vi "Error Log Example.vi"(3 "Send Error":bool, 4 "Erase":bool, 5 "Error Message":string="Error log message.", 6 "Show Console":bool, 7 "Error Level":T2(ring), 9 "Name":string(combo), 10 "Logger Display Format":T1=enum."PlainText.INI", 11 "Logger Name":string="Logger Example") -> ()   [LabVIEW 2018]
uses:
  <vilib>/BenjaminR/Error Log/Serializer/Type Defs/Display Format.ctl
  <vilib>/BenjaminR/Error Log/Handler.File.Text/Handler.File.Text.lvclass
  D:/Program Files (x86)/National Instruments/LabVIEW 2018/vi.lib/BenjaminR/Error Log/Handler/Handler.lvclass
  <vilib>/BenjaminR/Error Log/Handler.UserEvent.Console/Handler.UserEvent.Console.lvclass
  <userlib>/_OpenG.lib/file/file.llb/File Exists - Scalar__ogtk.vi
  <vilib>/BenjaminR/Error Log/Logger/Logger.lvclass
  <vilib>/BenjaminR/Error Log/Serializer/Serializer.lvlib
panel:
  in  "error in (no error)":errorcluster caption="错误输入（无错误）"
  in  "Error":errorcluster={"status"=TRUE, "code"=5000, "source"="My Error Code"}
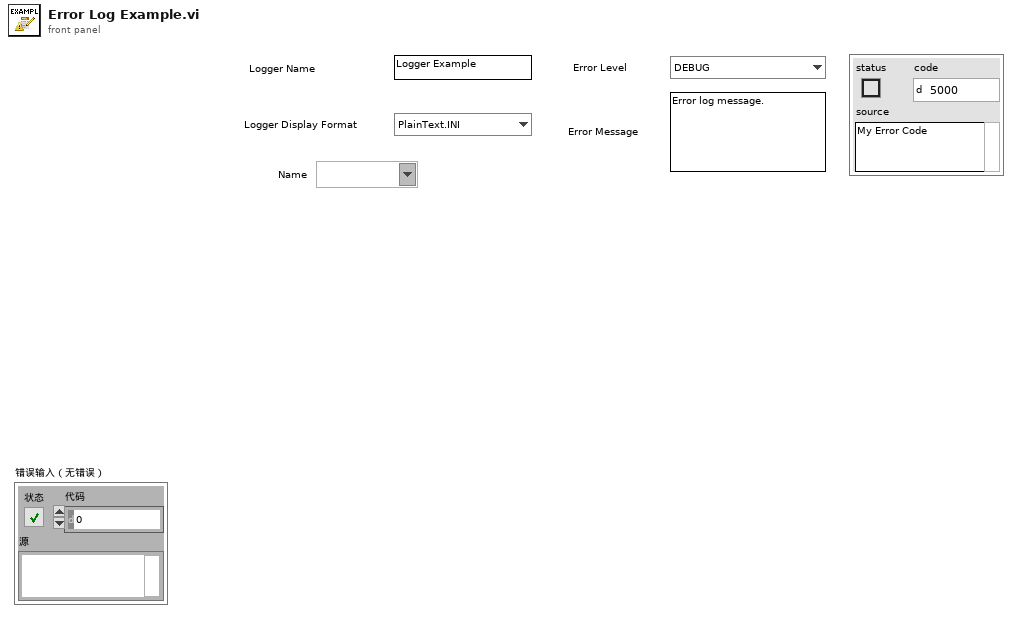
[diagram p1: front panel]
types:
  T1 = typedef "Serializer.lvlib/Display Format.ctl" = enum16{"PlainText", "PlainText.INI", "XML", "JSON"}
  T2 = enum16{"DEBUG", "INFO", "WARNING", "ERROR", "CRITICAL"}
  T3 = enum16{"open", "replace", "create", "open or create", "replace or create", "replace or create with confirmation"}
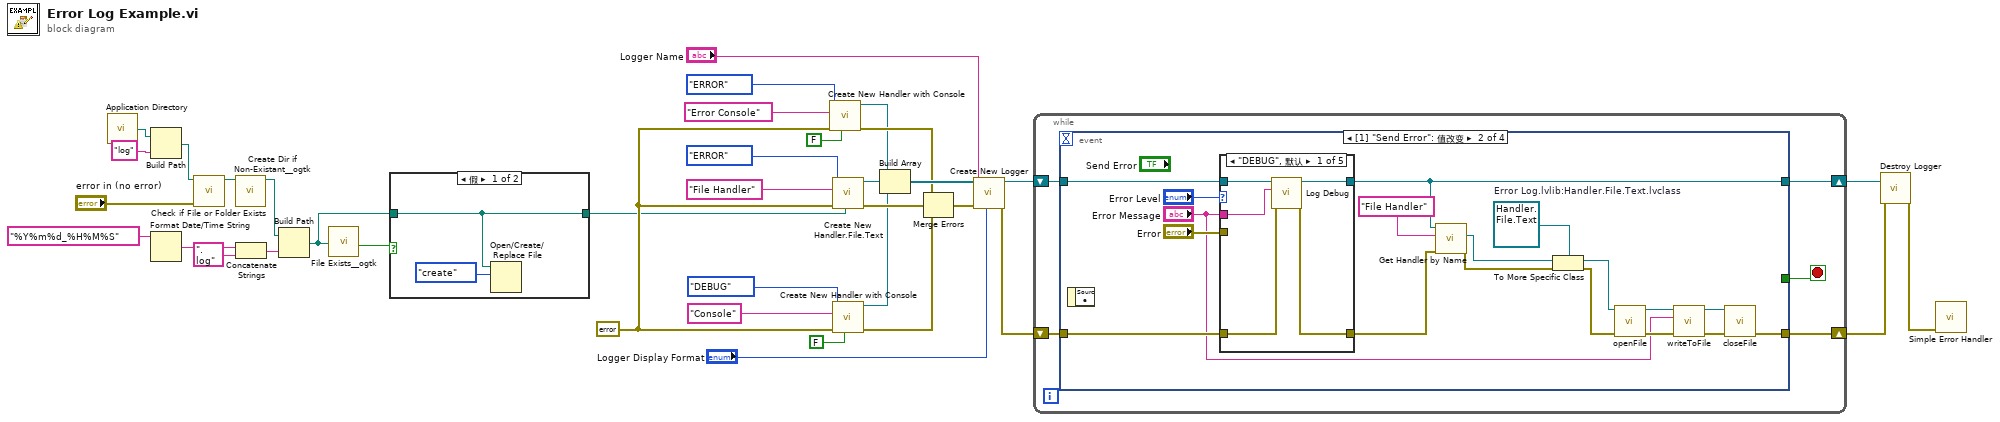
[diagram p0: block diagram]
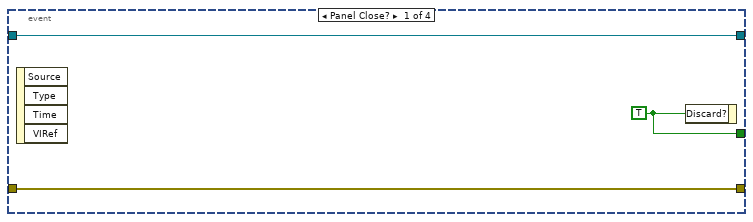
[diagram p3: hidden frame]
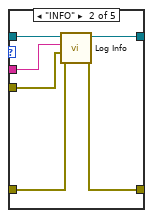
[diagram p4: hidden frame]
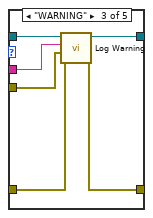
[diagram p5: hidden frame]
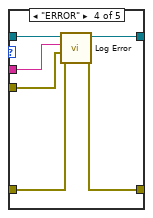
[diagram p6: hidden frame]
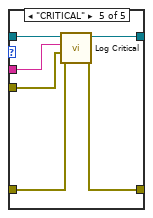
[diagram p7: hidden frame]
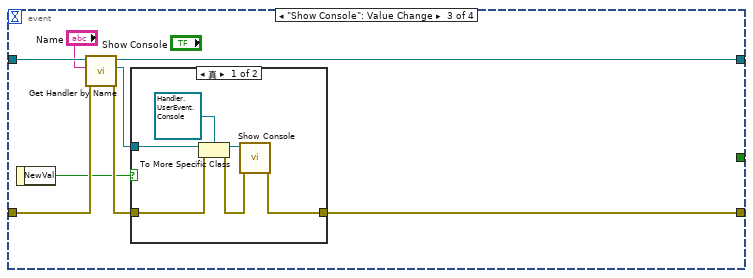
[diagram p8: hidden frame]
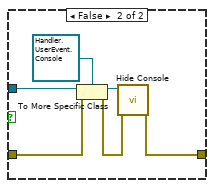
[diagram p9: hidden frame]
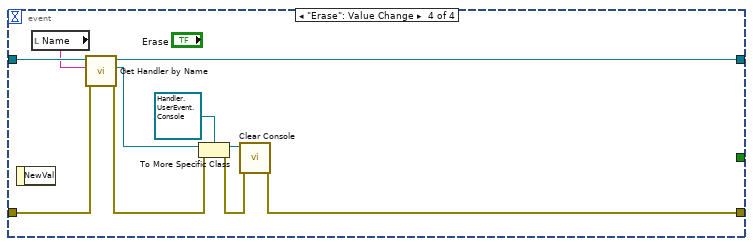
[diagram p10: hidden frame]
diagram:
  w16 = errorcluster {"status"=FALSE, "code"=0, "source"=""} ("error in (no error)")
  n1 = call <vilib>:"Application Directory.vi"() -> ("Application Directory"=w15:path)
  n2 = Build Path(base path=w15, name or relative path="log") -> (appended path=w13:path)
  n3 = Format Date/Time String(time format string (%c)="%Y%m%d_%H%M%S" ("时间格式字符串(%c)")) -> (date/time string=w8:string)  [unwired: 2 in]
  n4 = call <vilib>:"Check if File or Folder Exists.vi"("error in (no error)"="error in (no error)", "path"=w13) -> ("dup path"=w11:path)  [unwired: 7 in, 2 out]
  n5 = call <userlib>:"Create Dir if Non-Existant__ogtk.vi"("Directory Path"=w11) -> ("dup Directory Path"=w9:path)  [unwired: 8 in, 2 out]
  n6 = Concatenate Strings(w8, ".log" ("字符串")) -> (w6:string)
  n7 = Build Path(base path=w9, name or relative path=w6) -> (appended path=w4:path)
  n8 = call-poly <userlib>:"File Exists__ogtk.vi"("file path"=w4) -> ("exists"=w5:bool)  [unwired: 6 in, 1 out]
  n9 = case shown="假" w5 {
    tunnel: w4 -> [w38 w40]
    tunnel: [w38 w40] -> w1
    frame False {
      n10 = Open/Create/Replace File(file path (use dialog)=w38, operation (0:open)=T3."create" ("操作(0:open)")) -> ()  [unwired: 4 in, 3 out]
    }
    frame True {
    }
  }
  n11 = call <vilib>:"Create New Handler with Console.vi"("Show Console"=FALSE, "error in (no error)"=w16, "Name"="Error Console", "Level"=T2."ERROR") -> ("error out"=w20:errorcluster, "Handler.UserEvent.Console out"=w19:refnum<class "Handler.UserEvent.Console.lvclass">)  [unwired: 6 in]
  n12 = call <vilib>:"Create New Handler.File.Text.vi"("File Path"=w1, "error in (no error)"=w16, "Name"="File Handler", "Level"=T2."ERROR") -> ("error out"=w37:errorcluster, "Handler.File.Text out"=w36:refnum<class "Handler.File.Text.lvclass">)  [unwired: 6 in]
  n13 = call <vilib>:"Create New Handler with Console.vi"("Show Console"=FALSE, "error in (no error)"=w16, "Name"="Console", "Level"=T2."DEBUG") -> ("error out"=w27:errorcluster, "Handler.UserEvent.Console out"=w35:refnum<class "Handler.UserEvent.Console.lvclass">)  [unwired: 6 in]
  n14 = Build Array(w19, w36, w35) -> (w34:refnum<class "Handler.lvclass">[])
  n15 = Merge Errors(w20, w37, w27) -> (w33:errorcluster)
  n16 = call <vilib>:"Create New Logger.vi"("Display Format"="Logger Display Format", "error in (no error)"=w33, "Handlers"=w34, "Name"="Logger Name") -> ("error out"=w26:errorcluster, "Logger out"=w28:refnum<class "Logger.lvclass">)  [unwired: 6 in]
  n17 = while {
    shift-right: [w43] -> w25
    shift-left: w28 -> [w44]
    shift-right: [w41] -> w24
    shift-left: w26 -> [w42]
    stop <- w45 stop-if-true
    n18 = event shown="[1] \"Send Error\": 值改变" {
      selector: _ -> [_ _ _ _]
      dyn-events: _ -> [_ _ _ _]
      timeout: _ -> [_ _ _ _]
      tunnel: [w48 _ _ _] -> w45
      tunnel: w44 -> [w47 w66 w103 w125]
      tunnel: [w47 w62 w102 w124] -> w43
      tunnel: w42 -> [w46 w64 w101 w123]
      tunnel: [w46 w52 w98 w120] -> w41
      event Panel Close? {
        w48 = TRUE ("Discard?")
        n19 = event-data() -> ()  [unwired: 1 in, 4 out]
        n20 = event-data("Discard?"=w48) -> ()  [unwired: 1 in, 1 out]
      }
      event "Send Error": Value Change {
        w50 = refnum<class "Handler.File.Text.lvclass"> refnum  # Error Log.lvlib:Handler.File.Text.lvclass
        n21 = event-data() -> ()  [unwired: 1 in, 1 out]
        n22 = case shown="\"DEBUG\", 默认" "Error Level" {
          tunnel: w66 -> [w71 w77 w83 w89 w95]
          tunnel: [w70 w76 w82 w88 w94] -> w62
          tunnel: w64 -> [w69 w75 w81 w87 w93]
          tunnel: [w68 w74 w80 w86 w92] -> w61
          tunnel: "Error Message" -> [w67 w73 w79 w85 w91]
          tunnel: "Error" -> [_ w72 w78 w84 w90]
          frame "DEBUG", Default {
            n23 = call <vilib>:"Log Debug.vi"("error in (no error)"=w69, "Message"=w67, "Logger in"=w71) -> ("error out"=w68:errorcluster, "Logger out"=w70:refnum<class "Logger.lvclass">)  [unwired: 7 in]
          }
          frame "INFO" {
            n24 = call <vilib>:"Log Info.vi"("error in (no error)"=w75, "error"=w72, "Message"=w73, "Logger in"=w77) -> ("error out"=w74:errorcluster, "Logger out"=w76:refnum<class "Logger.lvclass">)  [unwired: 6 in]
          }
          frame "WARNING" {
            n25 = call <vilib>:"Log Warning.vi"("error in (no error)"=w81, "error"=w78, "Message"=w79, "Logger in"=w83) -> ("error out"=w80:errorcluster, "Logger out"=w82:refnum<class "Logger.lvclass">)  [unwired: 6 in]
          }
          frame "ERROR" {
            n26 = call <vilib>:"Log Error.vi"("error in (no error)"=w87, "error"=w84, "Message"=w85, "Logger in"=w89) -> ("error out"=w86:errorcluster, "Logger out"=w88:refnum<class "Logger.lvclass">)  [unwired: 6 in]
          }
          frame "CRITICAL" {
            n27 = call <vilib>:"Log Critical.vi"("error in (no error)"=w93, "error"=w90, "Message"=w91, "Logger in"=w95) -> ("error out"=w92:errorcluster, "Logger out"=w94:refnum<class "Logger.lvclass">)  [unwired: 6 in]
          }
        }
        n28 = call <vilib>:"Get Handler by Name.vi"("error in (no error)"=w61, "Handler Name"="File Handler" ("Name"), "Logger in"=w62) -> ("error out"=w54:errorcluster, "Handler"=w55:refnum<class "Handler.lvclass">)  [unwired: 6 in, 1 out]
        n29 = To More Specific Class(target class=w50, reference=w55, error in=w54) -> (specific class reference=w56:refnum<class "Handler.File.Text.lvclass">, error out=w53:errorcluster)
        n30 = call-dynamic "openFile.vi"("error in (no error)"=w53, "Handler.File.Text in"=w56) -> ("error out"=w59:errorcluster, "Handler.File.Text out"=w57:refnum<class "Handler.File.Text.lvclass">)  [unwired: 8 in]
        n31 = call-dynamic "writeToFile.vi"("error in (no error)"=w59, "New Record String"="Error Message", "Handler.File.Text in"=w57) -> ("error out"=w60:errorcluster, "Handler.File.Text out"=w58:refnum<class "Handler.File.Text.lvclass">)  [unwired: 7 in]
        n32 = call-dynamic "closeFile.vi"("error in (no error)"=w60, "Handler.File.Text in"=w58) -> ("error out"=w52:errorcluster)  [unwired: 8 in, 1 out]
      }
      event "Show Console": Value Change {
        n33 = event-data() -> ("NewVal"=w97:bool)  [unwired: 1 in]
        n34 = call <vilib>:"Get Handler by Name.vi"("error in (no error)"=w101, "Handler Name"="Name", "Logger in"=w103) -> ("error out"=w99:errorcluster, "Handler"=w100:refnum<class "Handler.lvclass">, "Logger out"=w102:refnum<class "Logger.lvclass">)  [unwired: 6 in]
        n35 = case shown="真" w97 {
          tunnel: w100 -> [w109 w115]
          tunnel: w99 -> [w106 w112]
          tunnel: [w104 w110] -> w98
          frame True {
            n36 = To More Specific Class(target class=refnum<class "Handler.UserEvent.Console.lvclass"> refnum ("Error Log.lvlib:Handler.UserEvent.Console.lvclass"), reference=w109, error in=w106) -> (specific class reference=w108:refnum<class "Handler.UserEvent.Console.lvclass">, error out=w105:errorcluster)
            n37 = call <vilib>:"Show Console.vi"("error in (no error)"=w105, "Handler.UserEvent.Console in"=w108) -> ("error out"=w104:errorcluster)  [unwired: 8 in, 1 out]
          }
          frame False {
            n38 = To More Specific Class(target class=refnum<class "Handler.UserEvent.Console.lvclass"> refnum ("Error Log.lvlib:Handler.UserEvent.Console.lvclass"), reference=w115, error in=w112) -> (specific class reference=w114:refnum<class "Handler.UserEvent.Console.lvclass">, error out=w111:errorcluster)
            n39 = call <vilib>:"Hide Console.vi"("error in (no error)"=w111, "Handler.UserEvent.Console in"=w114) -> ("error out"=w110:errorcluster)  [unwired: 8 in, 1 out]
          }
        }
      }
      event "Erase": Value Change {
        n40 = event-data() -> ()  [unwired: 1 in, 1 out]
        n41 = local read "Name"() -> (w116:string)
        n42 = call <vilib>:"Get Handler by Name.vi"("error in (no error)"=w123, "Handler Name"=w116, "Logger in"=w125) -> ("error out"=w121:errorcluster, "Handler"=w122:refnum<class "Handler.lvclass">, "Logger out"=w124:refnum<class "Logger.lvclass">)  [unwired: 6 in]
        n43 = To More Specific Class(target class=refnum<class "Handler.UserEvent.Console.lvclass"> refnum ("Error Log.lvlib:Handler.UserEvent.Console.lvclass"), reference=w122, error in=w121) -> (specific class reference=w119:refnum<class "Handler.UserEvent.Console.lvclass">, error out=w117:errorcluster)
        n44 = call <vilib>:"Clear Console.vi"("error in (no error)"=w117, "Handler.UserEvent.Console in"=w119) -> ("error out"=w120:errorcluster)  [unwired: 8 in, 1 out]
      }
    }
  }
  n45 = call <vilib>:"Destroy Logger.vi"("error in (no error)"=w24, "Logger in"=w25) -> ("error out"=w23:errorcluster)  [unwired: 8 in, 1 out]
  n46 = call <vilib>:"Simple Error Handler.vi"("error in (no error)"=w23) -> ()  [unwired: 4 in, 5 out]
